vi "Lang Set Image Page.vi"(8 "error in (no error)":errorcluster, 10 "Image":T1, 11 "Configuration Window in":refnum<class "Configuration Window.lvclass">) -> (0 "error out":errorcluster, 3 "Configuration Window out":refnum<class "Configuration Window.lvclass">)   [LabVIEW 2018, in "Configuration Window.lvlib" / "Configuration Window.lvclass"]
uses:
  Configuration Window.lvclass
  Framework/Framework/Const Lang CfgWnd Image.ctl
  Framework/Framework/Const Lang Property.ctl
  Configuration Window.lvclass/Configuration Window.ctl
  Framework/Framework/Framework.lvclass
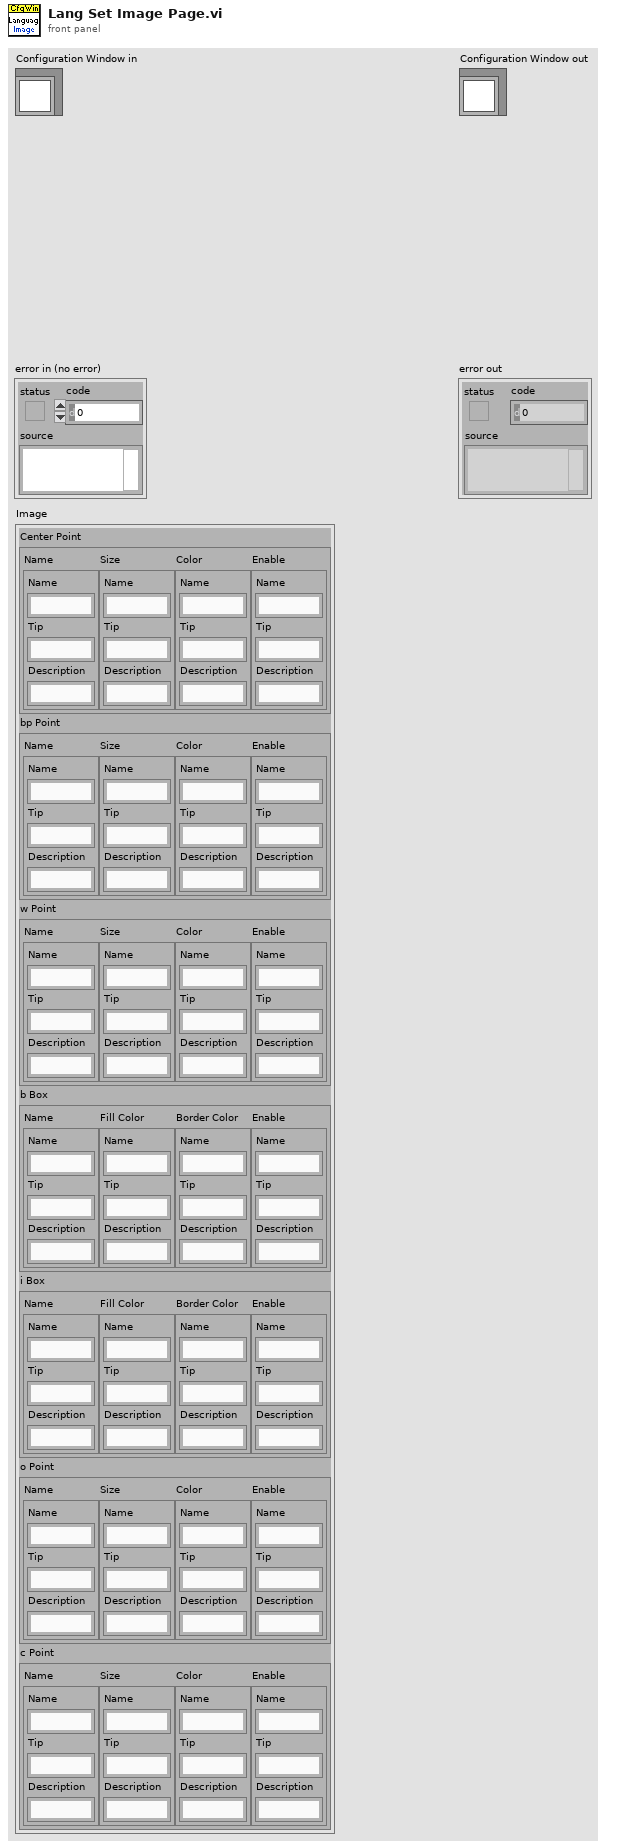
[diagram p1: front panel]
types:
  T1 = typedef "Framework.lvlib/Framework.lvclass/Const Lang CfgWnd Image.ctl" = cluster{"Center Point":cluster{"Name":T2, "Size":T2, "Color":T2, "Enable":T2}, "bp Point":cluster{"Name":T2, "Size":T2, "Color":T2, "Enable":T2}, "w Point":cluster{"Name":T2, "Size":T2, "Color":T2, "Enable":T2}, "b Box":cluster{"Name":T2, "Fill Color":T2, "Border Color":T2, "Enable":T2}, "i Box":cluster{"Name":T2, "Fill Color":T2, "Border Color":T2, "Enable":T2}, "o Point":cluster{"Name":T2, "Size":T2, "Color":T2, "Enable":T2}, "c Point":cluster{"Name":T2, "Size":T2, "Color":T2, "Enable":T2}}
  T2 = typedef "Framework.lvlib/Framework.lvclass/Const Lang Property.ctl" = cluster{"Name":string, "Tip":string, "Description":string}
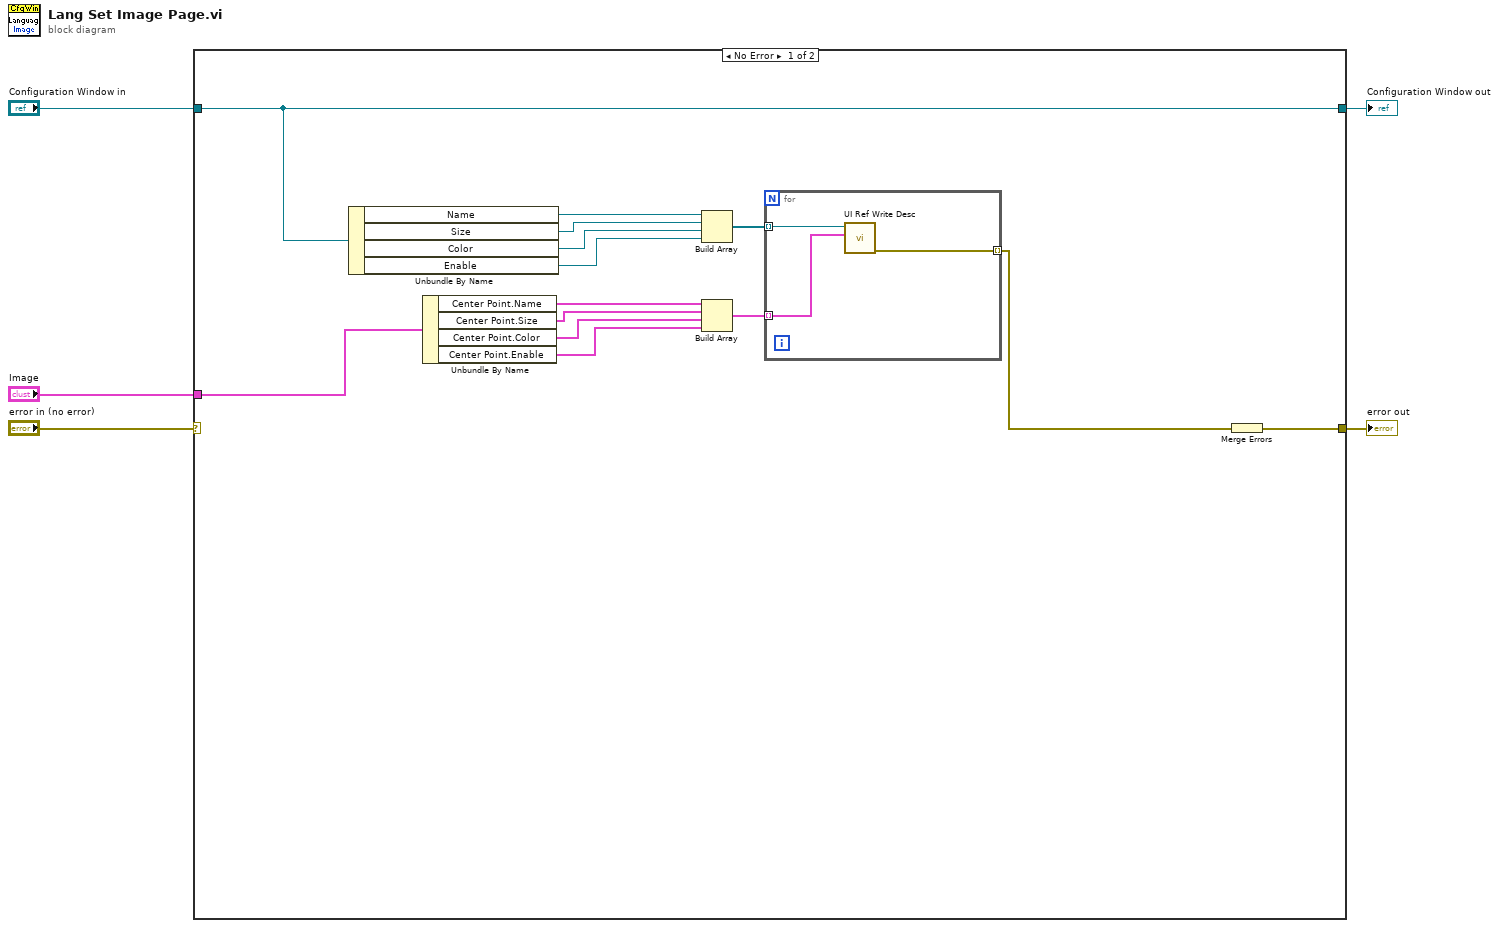
[diagram p0: block diagram]
diagram:
  n1 = case shown="No Error" "error in (no error)" {
    selector: "error in (no error)" -> [_ w24]
    tunnel: [w17 w24] -> w4
    tunnel: [w19 w23] -> w2
    tunnel: "Configuration Window in" -> [w19 w23]
    tunnel: "Image" -> [w12 _]
    frame No Error {
      n2 = Unbundle By Name(w19) -> ("Name"=w16:refnum<vi>, "Size"=w15:refnum<vi>, "Color"=w14:refnum<vi>, "Enable"=w13:refnum<vi>)
      n3 = Unbundle By Name(w12) -> ("Center Point.Name"=w11:T2, "Center Point.Size"=w10:T2, "Center Point.Color"=w9:T2, "Center Point.Enable"=w8:T2)
      n4 = Build Array(w16, w15, w14, w13) -> (w18:refnum<vi>[])
      n5 = Build Array(w11, w10, w9, w8) -> (w7:T2[])
      n6 = for {
        tunnel: w18 -> [w22] mode=indexing
        tunnel: w7 -> [w21] mode=indexing
        tunnel: [w20] -> w6 mode=indexing
        n7 = call "UI Ref Write Desc.vi"("UI Property"=w21, "UI Ref"=w22) -> ("error out"=w20:errorcluster)  [unwired: 9 in]
      }
      n8 = Merge Errors(w6) -> (w17:errorcluster)
    }
    frame Error {
    }
  }
  "error out" <- w4
  "Configuration Window out" <- w2
